vi "test_crc16.vi"() -> (3 "All Passed?":bool)   [LabVIEW 2021]
uses:
  src/hashlib.lvlib
panel:
  in  "Data in":string="123456789"
  out "CRC-16 out":T1(array[cluster]) {"CRC-16" format="%04x"}
  in  "CRC-16 Types":T2(array[cluster])=[{"Name"="CRC-16/CCITT-FALSE", "CRC16"=10673, "Initial"=65535, "Poly"=4129, "XorOut"=0, "ReflectIn"=FALSE, "ReflectOut"=FALSE}, {"Name"="CRC-16/ARC", "CRC16"=47933, "Initial"=0, "Poly"=32773, "XorOut"=0, "ReflectIn"=TRUE, "ReflectOut"=TRUE}, {"Name"="CRC-16/AUG-CCITT", "CRC16"=58828, "Initial"=7439, "Poly"=4129, "XorOut"=0, "ReflectIn"=FALSE, "ReflectOut"=FALSE}, {"Name"="CRC-16/BUYPASS", "CRC16"=65256, "Initial"=0, "Poly"=32773, "XorOut"=0, "ReflectIn"=FALSE, "ReflectOut"=FALSE}, {"Name"="CRC-16/CDMA2000", "CRC16"=19462, "Initial"=65535, "Poly"=51303, "XorOut"=0, "ReflectIn"=FALSE, "ReflectOut"=FALSE}, {"Name"="CRC-16/DDS-110", "CRC16"=40655, "Initial"=32781, "Poly"=32773, "XorOut"=0, "ReflectIn"=FALSE, "ReflectOut"=FALSE}, {"Name"="CRC-16/DECT-R", "CRC16"=126, "Initial"=0, "Poly"=1417, "XorOut"=1, "ReflectIn"=FALSE, "ReflectOut"=FALSE}, {"Name"="CRC-16/DECT-X", "CRC16"=127, "Initial"=0, "Poly"=1417, "XorOut"=0, "ReflectIn"=FALSE, "ReflectOut"=FALSE}, {"Name"="CRC-16/DNP", "CRC16"=60034, "Initial"=0, "Poly"=15717, "XorOut"=65535, "ReflectIn"=TRUE, "ReflectOut"=TRUE}, {"Name"="CRC-16/EN-13757", "CRC16"=49847, "Initial"=0, "Poly"=15717, "XorOut"=65535, "ReflectIn"=FALSE, "ReflectOut"=FALSE}, {"Name"="CRC-16/GENIBUS", "CRC16"=54862, "Initial"=65535, "Poly"=4129, "XorOut"=65535, "ReflectIn"=FALSE, "ReflectOut"=FALSE}, {"Name"="CRC-16/MAXIM", "CRC16"=17602, "Initial"=0, "Poly"=32773, "XorOut"=65535, "ReflectIn"=TRUE, "ReflectOut"=TRUE}, {"Name"="CRC-16/MCRF4XX", "CRC16"=28561, "Initial"=65535, "Poly"=4129, "XorOut"=0, "ReflectIn"=TRUE, "ReflectOut"=TRUE}, {"Name"="CRC-16/RIELLO", "CRC16"=25552, "Initial"=45738, "Poly"=4129, "XorOut"=0, "ReflectIn"=TRUE, "ReflectOut"=TRUE}, {"Name"="CRC-16/T10-DIF", "CRC16"=53467, "Initial"=0, "Poly"=35767, "XorOut"=0, "ReflectIn"=FALSE, "ReflectOut"=FALSE}, {"Name"="CRC-16/TELEDISK", "CRC16"=4019, "Initial"=0, "Poly"=41111, "XorOut"=0, "ReflectIn"=FALSE, "ReflectOut"=FALSE}, {"Name"="CRC-16/TMS37157", "CRC16"=9905, "Initial"=35308, "Poly"=4129, "XorOut"=0, "ReflectIn"=TRUE, "ReflectOut"=TRUE}, {"Name"="CRC-16/USB", "CRC16"=46280, "Initial"=65535, "Poly"=32773, "XorOut"=65535, "ReflectIn"=TRUE, "ReflectOut"=TRUE}, {"Name"="CRC-16/A", "CRC16"=48901, "Initial"=50886, "Poly"=4129, "XorOut"=0, "ReflectIn"=TRUE, "ReflectOut"=TRUE}, {"Name"="CRC-16/KERMIT", "CRC16"=8585, "Initial"=0, "Poly"=4129, "XorOut"=0, "ReflectIn"=TRUE, "ReflectOut"=TRUE}, {"Name"="CRC-16/MODBUS", "CRC16"=19255, "Initial"=65535, "Poly"=32773, "XorOut"=0, "ReflectIn"=TRUE, "ReflectOut"=TRUE}, {"Name"="CRC-16/X-25", "CRC16"=36974, "Initial"=65535, "Poly"=4129, "XorOut"=65535, "ReflectIn"=TRUE, "ReflectOut"=TRUE}, {"Name"="CRC-16/XMODEM", "CRC16"=12739, "Initial"=0, "Poly"=4129, "XorOut"=0, "ReflectIn"=FALSE, "ReflectOut"=FALSE}] {"XorOut" format="%04x"; "CRC16" format="%04x"; "Poly" format="%04x"; "Initial" format="%04x"}
  # "https://crccalc.com/"
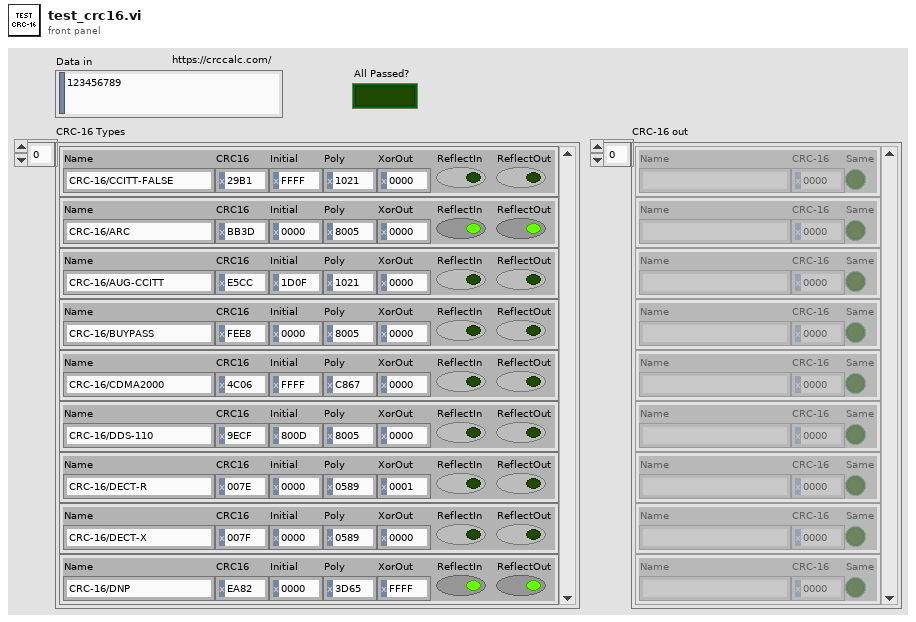
[diagram p1: front panel]
types:
  T1 = cluster{"Name":string, "CRC-16":u16, "Same":bool}[]
  T2 = cluster{"Name":string, "CRC16":u16, "Initial":u16, "Poly":u16, "XorOut":u16, "ReflectIn":bool, "ReflectOut":bool}[]
  T3 = cluster{"Name":string, "CRC-16":u16, "Same":bool}
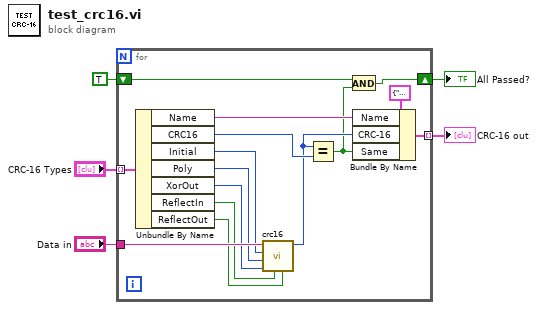
[diagram p0: block diagram]
diagram:
  n1 = for {
    tunnel: "Data in" -> [w20]
    tunnel: "CRC-16 Types" -> [w19] mode=indexing
    tunnel: [w16] -> w3 mode=indexing
    shift-right: [w11] -> w1
    shift-left: TRUE -> [w13]
    n2 = Unbundle By Name(w19) -> ("Name"=w17:string, "CRC16"=w15:u16, "Initial"=w10:u16, "Poly"=w9:u16, "XorOut"=w8:u16, "ReflectIn"=w7:bool, "ReflectOut"=w6:bool)
    n3 = call "crc16.vi"("Reflect Output? (F)"=w6, "Reflect Input? (F)"=w7, "Xor Out (0x0000)"=w8, "Poly (0x8005)"=w9, "Init (0x0000)"=w10, "Data in"=w20) -> ("CRC-16"=w14:u16)  [unwired: 5 in]
    n4 = Equal?(x=w14, y=w15) -> (x = y?=w12:bool)
    n5 = And(x=w13, y=w12) -> (x .and. y?=w11:bool)
    n6 = Bundle By Name(cluster=T3 {"Name"="", "CRC-16"=0, "Same"=FALSE} ("CRC-16"), "Name"=w17, "CRC-16"=w14, "Same"=w12) -> (w16:T3)
  }
  "CRC-16 out" <- w3
  "All Passed?" <- w1
